vi "DEPRACATE Execute (sync).vi"(8 "error in (no error)":errorcluster, 10 "command":string, 11 "PQ Connection in":refnum<class "PQ Connection.lvclass">) -> (0 "error out":errorcluster, 1 "PQ Result  out":refnum<class "PQ Result.lvclass">, 2 "Number of Rows":i32, 3 "PQ Connection out":refnum<class "PQ Connection.lvclass">, 4 "PGresult":T1)   [LabVIEW 2015, in "PQ Connection.lvclass"]
uses:
  PQ Connection.lvclass
  Result/PQ Result.lvclass
  <vilib>/LAVA/libpq/Types/PGresult.ctl
  PQ Connection.lvclass/PQ Connection.ctl
  Result/PQ Result.lvclass/PQ Result.ctl
  libpq.dll
  <vilib>/LAVA/libpq/__lava_libpq.lvlib
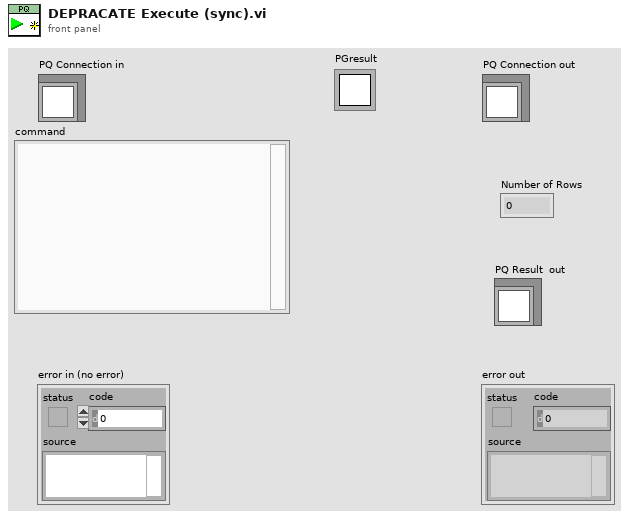
[diagram p1: front panel]
types:
  T1 = typedef "__lava_libpq.lvlib/PGresult.ctl" = refnum<k1>
  T2 = typedef "Result Status.ctl" = enum32{"PGRES_EMPTY_QUERY", "PGRES_COMMAND_OK", "PGRES_TUPLES_OK", "PGRES_COPY_OUT", "PGRES_COPY_IN", "PGRES_BAD_RESPONSE", "PGRES_NONFATAL_ERROR", "PGRES_FATAL_ERROR", "PGRES_COPY_BOTH", "PGRES_SINGLE_TUPLE"}
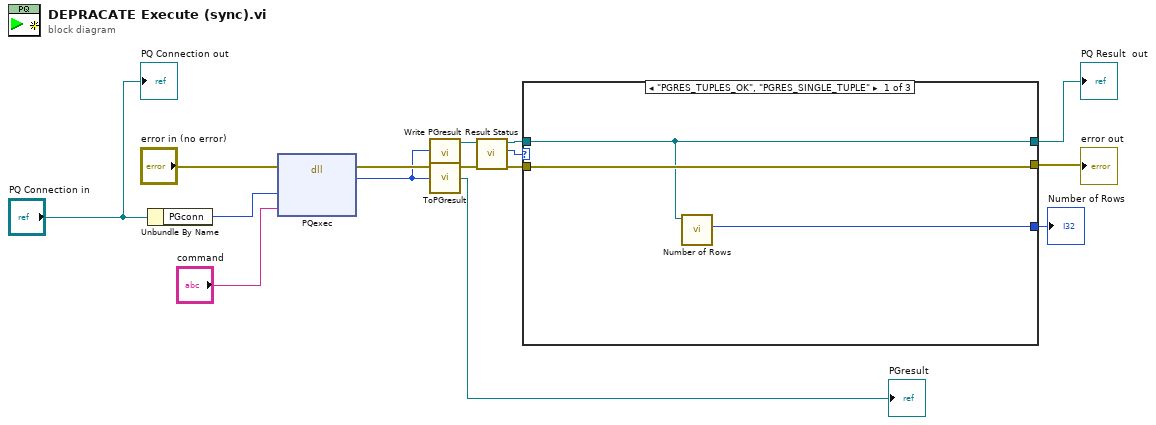
[diagram p0: block diagram]
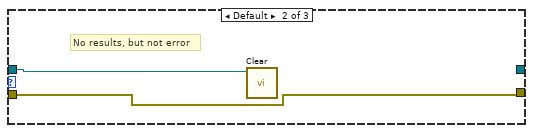
[diagram p2: hidden frame]
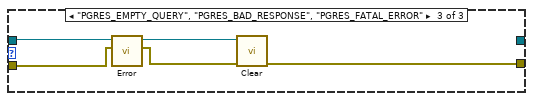
[diagram p3: hidden frame]
diagram:
  n1 = Unbundle By Name("PQ Connection in") -> ("PGconn"=w13:u32)
  n2 = dll-call lib="C:/PQ/Connection/libpq.dll" fn="PQexec"(error in="error in (no error)", "PGconn"=w13, "command"="command") -> (error out=w12:errorcluster, "PQresult"=w9:u32)  [unwired: 4 in, 1 out]
  n3 = call "Write PGresult.vi"("error in (no error)"=w12, "PGresult"=w9) -> ("error out"=w7:errorcluster, "PQ Result  out"=w11:refnum<class "PQ Result.lvclass">)  [unwired: 8 in]
  n4 = call <vilib>:"ToPGresult.vi"("PGconn_ptr"=w9) -> ("PGresult"=→"PGresult":T1)
  n5 = call "Result Status.vi"("error in (no error)"=w7, "PQ Result in"=w11) -> ("error out"=w3:errorcluster, "Result Status"=w6:T2, "PQ Result out"=w4:refnum<class "PQ Result.lvclass">)  [unwired: 7 in]
  n6 = case shown="\"PGRES_TUPLES_OK\", \"PGRES_SINGLE_TUPLE\"" w6 {
    tunnel: [w17 _ _] -> w5
    tunnel: w4 -> [w17 w20 w25]
    tunnel: w3 -> [w18 w19 w24]
    tunnel: [w18 w19 w22] -> w2
    tunnel: [w16 _ _] -> w1
    frame "PGRES_TUPLES_OK", "PGRES_SINGLE_TUPLE" {
      n7 = call "Number of Rows.vi"("PQ Result in"=w17) -> ("Number of Rows"=w16:i32)  [unwired: 8 in, 2 out]
    }
    frame Default {
      # "No results, but not error"
      n8 = call "Clear.vi"("PQ Result  in"=w20) -> ()  [unwired: 10 in, 1 out]
    }
    frame "PGRES_EMPTY_QUERY", "PGRES_BAD_RESPONSE", "PGRES_FATAL_ERROR" {
      n9 = call "Error.vi"("error in (no error)"=w24, "PQ Result  In"=w25) -> ("error out"=w23:errorcluster, "PQ Result"=w21:refnum<class "PQ Result.lvclass">)  [unwired: 8 in]
      n10 = call "Clear.vi"("error in (no error)"=w23, "PQ Result  in"=w21) -> ("error out"=w22:errorcluster)  [unwired: 9 in]
    }
  }
  "error out" <- w2
  "PQ Result  out" <- w5
  "Number of Rows" <- w1
  "PQ Connection out" <- "PQ Connection in"
